vi "Boolean to JSON element.vi"(7 "prefix":string, 10 "boolean":bool, 11 "keyword":string) -> (2 "JSON last element":string, 3 "JSON element":string)   [LabVIEW 2018]
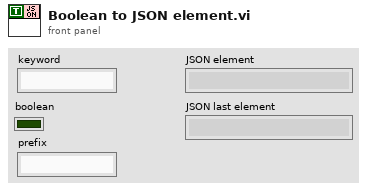
[diagram p1: front panel]
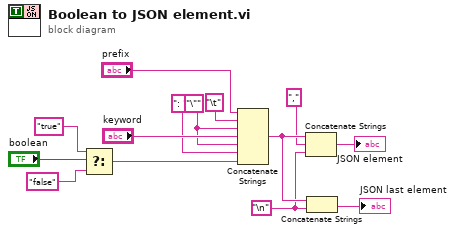
[diagram p0: block diagram]
diagram:
  w3 = "\n"
  w12 = "\""
  n1 = Select(t="true", s="boolean", f="false") -> (s? t:f=w8:string)
  n2 = Concatenate Strings("prefix", "\t", w12, "keyword", w12, ": ", w8) -> (w5:string)
  n3 = Concatenate Strings(w5, ",", w3) -> (→"JSON element":string)
  n4 = Concatenate Strings(w5, w3) -> (→"JSON last element":string)
